vi "SV_Control_Json.vi"() -> ()   [LabVIEW 2026]
uses:
  <vilib>/Instr/_visa.llb/VISA Configure Serial Port (Instr).vi
panel:
  out "CONFIRMATION":string
  out "JSON command cluster":string
  in  "ESP32":refnum<visa-resource-name>
  in  "stop":bool
  in  "Relay \n1":bool
  in  "Relay \n2":bool
  in  "Relay \n3":bool
  in  "Relay \n4":bool
  out "LED 1":bool
  out "LED 2":bool
  out "LED 3":bool
  out "LED 4":bool
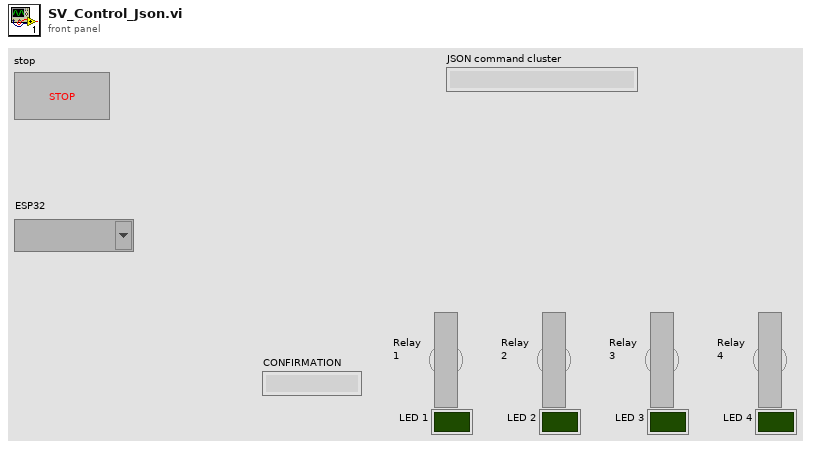
[diagram p1: front panel]
types:
  T1 = cluster{"SV1":i32, "SV2":i32, "SV3":i32, "SV4":i32}
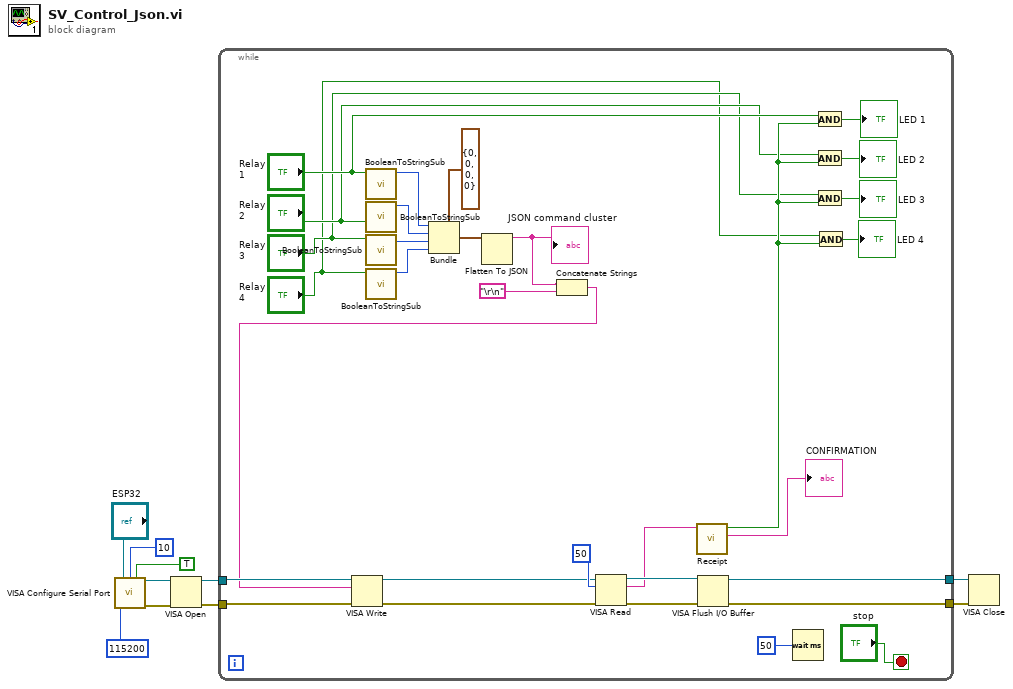
[diagram p0: block diagram]
diagram:
  n1 = call-poly "VISA Configure Serial Port"("VISA resource name"="ESP32", "termination char\n(0xA = '\\n' = LF)"=u8 10 ("termination char\n(0xA = '\\n' = LF)"), "Enable Termination\nChar (T)"=TRUE ("Enable Termination\nChar (T)"), "baud rate (9600)"=u32 115200) -> ("VISA resource name out"=w8:refnum<visa-resource-name>, "error out"=w7:errorcluster)  [unwired: 10 in]
  n2 = VISA Open(error in (no error)=w7, VISA resource name=w8) -> (VISA resource name=w5:refnum<visa-resource-name>, error out=w6:errorcluster)  [unwired: 3 in]
  n3 = while {
    tunnel: w6 -> [w38]
    tunnel: w5 -> [w39]
    tunnel: [w35] -> w4
    tunnel: [w34] -> w3
    stop <- "stop" stop-if-true
    n4 = call "BooleanToStringSub.vi"("Relay Switch"="Relay \n1") -> ("Numeric"=w30:i32)  [unwired: 10 in]
    n5 = call "BooleanToStringSub.vi"("Relay Switch"="Relay \n2") -> ("Numeric"=w29:i32)  [unwired: 10 in]
    n6 = call "BooleanToStringSub.vi"("Relay Switch"="Relay \n3") -> ("Numeric"=w28:i32)  [unwired: 10 in]
    n7 = call "BooleanToStringSub.vi"("Relay Switch"="Relay \n4") -> ("Numeric"=w27:i32)  [unwired: 10 in]
    n8 = Bundle(cluster=T1 {"SV1"=0, "SV2"=0, "SV3"=0, "SV4"=0}, "SV1"=w30, "SV2"=w29, "SV3"=w28, "SV4"=w27) -> (w22:T1)
    n9 = Flatten To JSON(anything=w22) -> (JSON string=w26:string)  [unwired: 2 in, 1 out]
    "JSON command cluster" <- w26
    n10 = Concatenate Strings(w26, "\r\n") -> (w24:string)
    n11 = VISA Write(VISA resource name=w39, write buffer=w24, error in (no error)=w38) -> (VISA resource name out=w32:refnum<visa-resource-name>, error out=w31:errorcluster)  [unwired: 1 out]
    n12 = VISA Read(VISA resource name=w32, byte count=u32 50, error in (no error)=w31) -> (VISA resource name out=w37:refnum<visa-resource-name>, read buffer=w21:string, error out=w36:errorcluster)  [unwired: 1 out]
    n13 = call "Receipt.vi"("read buffer"=w21) -> ("String"=→"CONFIRMATION":string, "Boolean"=w15:bool)  [unwired: 9 in]
    n14 = VISA Flush I/O Buffer(VISA resource name=w37, error in (no error)=w36) -> (VISA resource name out=w35:refnum<visa-resource-name>, error out=w34:errorcluster)  [unwired: 1 in]
    n15 = Wait (ms)(milliseconds to wait=u32 50) -> ()  [unwired: 1 out]
    n16 = And(x="Relay \n1", y=w15) -> (x .and. y?=→"LED 1":bool)
    n17 = And(x="Relay \n2", y=w15) -> (x .and. y?=→"LED 2":bool)
    n18 = And(x="Relay \n3", y=w15) -> (x .and. y?=→"LED 3":bool)
    n19 = And(x="Relay \n4", y=w15) -> (x .and. y?=→"LED 4":bool)
  }
  n20 = VISA Close(VISA resource name=w4, error in (no error)=w3) -> ()  [unwired: 1 out]
